vi "AlarmInsert.vi"(6 "提示":string="正常", 7 "takesTime":string, 9 "级别":string="10", 10 "类型":string="装配步骤", 11 "消息名":string) -> ()   [LabVIEW 2012]
uses:
  resultShow.vi
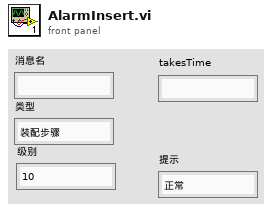
[diagram p1: front panel]
types:
  T1 = cluster{"takesTime":refnum<vi>, "userStatus":refnum<vi>, "userName":refnum<vi>, "connectionMode":refnum<vi>, "productsName":refnum<vi>, "rigStatus":refnum<vi>, "管柱码":refnum<vi>, "电机码":refnum<vi>, "控制器码":refnum<vi>, "rigStatus 2":refnum<vi>}
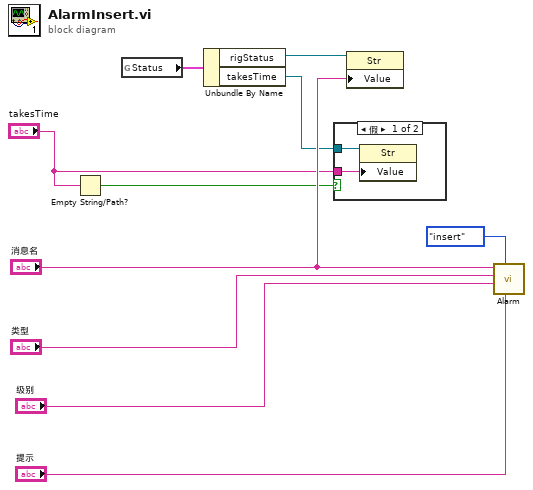
[diagram p0: block diagram]
diagram:
  n1 = Empty String/Path?(string/path="takesTime") -> (empty?=w1:bool)
  n2 = global read "resultShow.vi" "Status"() -> (w10:T1)
  n3 = Unbundle By Name(w10) -> ("rigStatus"=w9:refnum<vi>, "takesTime"=w3:refnum<vi>)
  n4 = case shown="假" w1 {
    tunnel: w3 -> [w12 _]
    tunnel: "takesTime" -> [w11 _]
    frame False {
      n5 = property class="Str"(reference=w12, "Value"=w11) -> ()  [unwired: 1 in, 2 out]
    }
    frame True {
    }
  }
  n6 = property class="Str"(reference=w9, "Value"="消息名") -> ()  [unwired: 1 in, 2 out]
  n7 = call "Alarm.vi"("提示"="提示", "模式"=enum16{"select", "insert", "update", "delete"}."insert", "级别"="级别", "类型"="类型", "消息名"="消息名") -> ()  [unwired: 6 in, 1 out]
